vi "OAT Easy Resample Order Tracking (Digital Tach).vi"(0 "scaled signal [EU]":waveform(dbl)={"t0"=timestamp(0 s since 1904-01-01), "dt"=0.0, "Y"=[]}, 1 "reset? (True)":bool=TRUE, 5 "orders (1.0)":dbl[](array[numeric])=[1.0] format="%.2f", 7 "digital tach info":T3={"tacho counts"=[], "counter timebase [Hz]"=20000000.0, "counter task type"=enum."event counting", "counter digit (32)"=32}, 9 "pulse/revolution (1)":i32=1, 11 "error in (no error)":errorcluster, 12 "X axis selection":u16(ring)=2 items=["Time", "Revolution", "RPM"], 13 "phase setting":T1, 14 "bandwidth":dbl=-1.0 format="%.2f") -> (3 "samples/rev":dbl format="%.2f", 4 "magnitudes (RMS)":cluster{"X":dbl[], "Y":dbl[]}[](array[cluster]) {"Y" format="%.2f"; "X" format="%.2f"}, 6 "phase lags":cluster{"X":dbl[], "Y":dbl[]}[](array[cluster]) {"Y" format="%.2f"; "X" format="%.2f"}, 10 "unit labels":T2, 15 "error out":errorcluster)   [LabVIEW 2017]
doc: "Computes magnitudes and phase lags for the designated orders for <B>scaled signal [EU]</B>. You can use this polymorphic VI to perform order tracking with resampling for an analog tachometer signal or a digital tachometer signal. The data type you wire to the <B>analog tach signal</B> input determines the polymorphic instance to use."
uses:
  <vilib>/addons/Sound and Vibration/Order Analysis/Tach Process/SubVIs/digital tach info.ctl
  <vilib>/addons/Sound and Vibration/Order Analysis/Tach Process/SubVIs/speed profile.ctl
  <vilib>/addons/Sound and Vibration/Order Analysis/Backward Compatibility/OAT Track Orders in Resampled Signal (Single Channel).vi
  <vilib>/addons/Sound and Vibration/Order Analysis/Backward Compatibility/OAT Resample Waveform (Single Channel).vi
  <vilib>/addons/Sound and Vibration/Order Analysis/Tach Process/SoundVib_TachProcess.lvlib
panel:
  # "OAT Easy Resample Order Tracking (Digital Tach)"
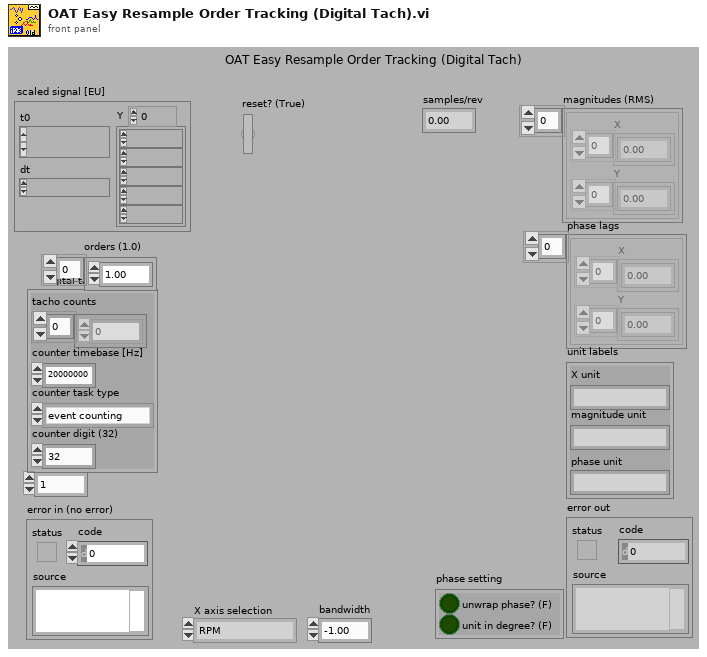
[diagram p1: front panel]
types:
  T1 = cluster{"unwrap phase? (F)":bool, "unit in degree? (F)":bool}
  T2 = cluster{"X unit":string, "magnitude unit":string, "phase unit":string}
  T3 = typedef "SoundVib_TachProcess.lvlib/digital tach info.ctl" = cluster{"tacho counts":i64[], "counter timebase [Hz]":dbl, "counter task type":enum16{"period measurement", "event counting"}, "counter digit (32)":i32}
  T4 = typedef "SoundVib_TachProcess.lvlib/speed profile.ctl" = cluster{"time [s]":dbl[], "speed [RPM]":dbl[]}
  T5 = typedef "svc_Channel Info.ctl" = cluster{"sensor sensitivity":dbl, "engineering units":T6, "dB reference":dbl, "custom label":string, "weighting filter":T7, "pregain":dbl}
  T6 = typedef "svc_Engineering Units Text Ring.ctl" = u16
  T7 = typedef "svc_Weighting Filter Text Ring.ctl" = u16
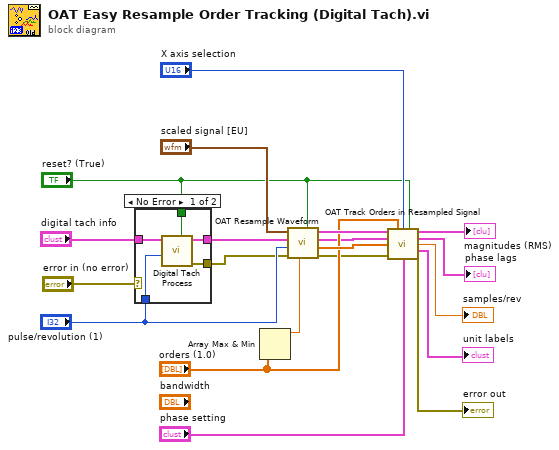
[diagram p0: block diagram]
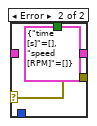
[diagram p2: hidden frame]
diagram:
  n1 = case shown="No Error" "error in (no error)" {
    selector: "error in (no error)" -> [_ w26]
    tunnel: "digital tach info" -> [w25 _]
    tunnel: [w24 T4 {"time [s]"=[], "speed [RPM]"=[]} ("speed profile")] -> w11
    tunnel: "pulse/revolution (1)" -> [w23 _]
    tunnel: "reset? (True)" -> [w22 _]
    tunnel: [w21 w26] -> w5
    frame No Error {
      n2 = call <vilib>:"Digital Tach Process.vi"("reset? (True)"=w22, "pulse/revolution (1)"=w23, "digital tach info"=w25) -> ("error out"=w21:errorcluster, "speed profile"=w24:T4)  [unwired: 6 in, 1 out]
    }
    frame Error {
    }
  }
  n3 = Array Max & Min(array="orders (1.0)") -> (max value=w6:dbl)  [unwired: 3 out]
  n4 = call-poly <vilib>:"OAT Resample Waveform.vi"("reset? (True)"="reset? (True)", "max order (auto)"=w6, "error in (no error)"=w5, "pulse/revolution (1)"="pulse/revolution (1)", "speed profile"=w11, "scaled signal [EU]"="scaled signal [EU]") -> ("error out"=w4:errorcluster, "interpolated pulse positions"=w12:dbl[], "channel info"=w7:T5, "resampled signal"=w18:cluster{"r0":dbl, "dr":dbl, "Y":dbl[]})  [unwired: 2 in]
  n5 = call-poly <vilib>:"OAT Track Orders in Resampled Signal.vi"("resampled signal"=w18, "orders (1.0)"="orders (1.0)", "X axis selection"="X axis selection", "reset? (True)"="reset? (True)", "channel info"=w7, "time instant"=w12, "error in (no error)"=w4, "phase setting"="phase setting") -> ("magnitudes (RMS)"=→"magnitudes (RMS)":cluster{"X":dbl[], "Y":dbl[]}[], "phase lags"=→"phase lags":cluster{"X":dbl[], "Y":dbl[]}[], "samples/rev"=→"samples/rev":dbl, "unit labels"=→"unit labels":T2, "error out"=→"error out":errorcluster)  [unwired: 3 in]
